vi "View Cooldown Results.vi"(6 "Temperature":dbl, 7 "OSC Configuration":T1(array[cluster]), 9 "Results":dbl[][](array[numeric]), 10 "Lockins":u16[](array[numeric]), 11 "Boolean":bool) -> (3 "Array":cluster{"Y":dbl[], "Y":dbl[]}[][](array[cluster]))   [LabVIEW 2013]
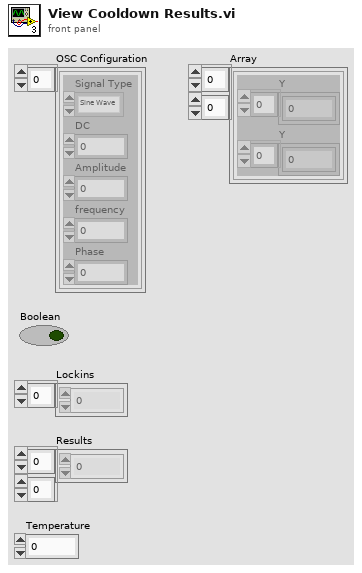
[diagram p1: front panel]
types:
  T1 = cluster{"Signal Type":enum16{"Sine Wave", "Triangle Wave", "Square Wave", "Sawtooth Wave"}, "DC":dbl, "Amplitude":dbl, "frequency":dbl, "Phase":dbl}[]
  T2 = cluster{"Signal Type":enum16{"Sine Wave", "Triangle Wave", "Square Wave", "Sawtooth Wave"}, "DC":dbl, "Amplitude":dbl, "frequency":dbl, "Phase":dbl}
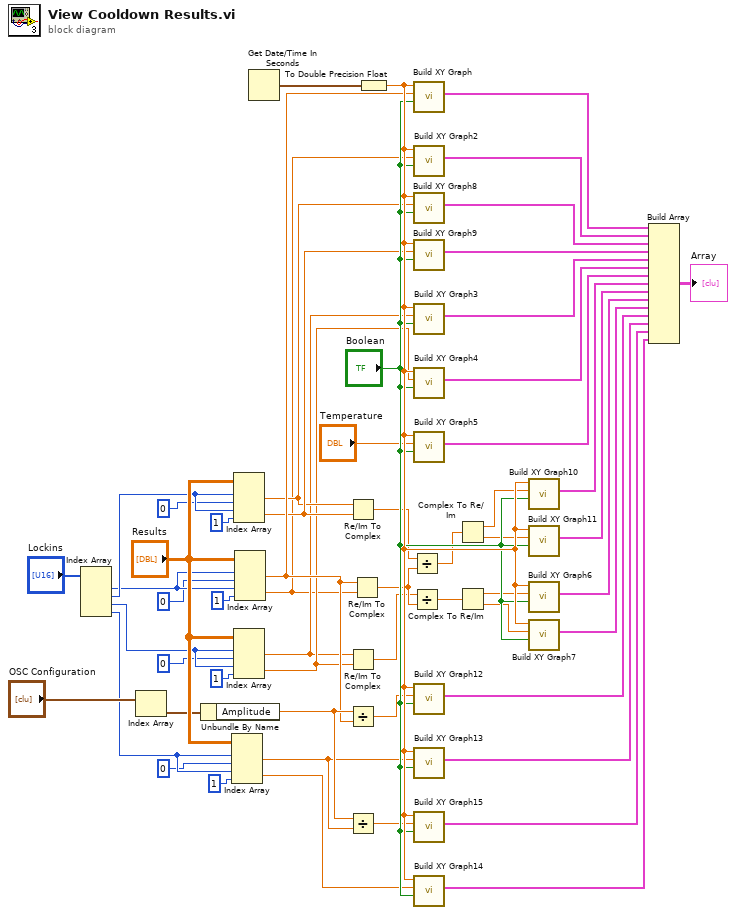
[diagram p0: block diagram]
diagram:
  n1 = Index Array(array="Lockins") -> (element #1=w31:u16, element #2=w32:u16, element #3=w33:u16, element #4=w30:u16)  [unwired: 4 in]
  n2 = Index Array(array="OSC Configuration") -> (element=w37:T2)  [unwired: 1 in]
  n3 = Unbundle By Name(w37) -> ("Amplitude"=w38:dbl)
  n4 = Index Array(array="Results", index (row) #1=w30, index (col) #1=0 ("disabled index (col)"), index (row) #2=w30, index (col) #2=1 ("disabled index (col)")) -> (element #1=w27:dbl, element #2=w26:dbl)
  n5 = Index Array(array="Results", index (row) #1=w32, index (col) #1=0 ("disabled index (col)"), index (row) #2=w32, index (col) #2=1 ("disabled index (col)")) -> (element #1=w15:dbl, element #2=w16:dbl)
  n6 = Index Array(array="Results", index (row) #1=w33, index (col) #1=0 ("disabled index (col)"), index (row) #2=w33, index (col) #2=1 ("disabled index (col)")) -> (element #1=w6:dbl, element #2=w7:dbl)
  n7 = Index Array(array="Results", index (row) #1=w31, index (col) #1=0 ("disabled index (col)"), index (row) #2=w31, index (col) #2=1 ("disabled index (col)")) -> (element #1=w22:dbl, element #2=w5:dbl)
  n8 = Get Date/Time In Seconds() -> (seconds since 1Jan1904=w34:timestamp)
  n9 = Re/Im To Complex(1:w16, 2:w15) -> (0:w17:cdb)
  n10 = Re/Im To Complex(1:w7, 2:w6) -> (0:w8:cdb)
  n11 = Divide(x=w38, y=w22) -> (x/y=w23:dbl)
  n12 = Divide(x=w38, y=w27) -> (x/y=w28:dbl)
  n13 = Re/Im To Complex(1:w5, 2:w22) -> (0:w18:cdb)
  n14 = To Double Precision Float(number=w34) -> (double precision float=w35:dbl)
  n15 = Divide(x=w17, y=w18) -> (x/y=w19:cdb)
  n16 = Divide(x=w8, y=w18) -> (x/y=w9:cdb)
  n17 = call "Build XY Graph"("Reset"="Boolean", "Y Input"=w22, "X Input"=w35) -> ("XY Graph"=w42:cluster{"Y":dbl[], "Y":dbl[]}[])  [unwired: 2 in, 6 out]
  n18 = call "Build XY Graph2"("Reset"="Boolean", "Y Input"=w5, "X Input"=w35) -> ("XY Graph"=w43:cluster{"Y":dbl[], "Y":dbl[]}[])  [unwired: 2 in, 6 out]
  n19 = call "Build XY Graph8"("Reset"="Boolean", "Y Input"=w15, "X Input"=w35) -> ("XY Graph"=w44:cluster{"Y":dbl[], "Y":dbl[]}[])  [unwired: 2 in, 6 out]
  n20 = call "Build XY Graph9"("Reset"="Boolean", "Y Input"=w16, "X Input"=w35) -> ("XY Graph"=w45:cluster{"Y":dbl[], "Y":dbl[]}[])  [unwired: 2 in, 6 out]
  n21 = call "Build XY Graph3"("Reset"="Boolean", "Y Input"=w6, "X Input"=w35) -> ("XY Graph"=w46:cluster{"Y":dbl[], "Y":dbl[]}[])  [unwired: 2 in, 6 out]
  n22 = call "Build XY Graph4"("Reset"="Boolean", "Y Input"=w7, "X Input"=w35) -> ("XY Graph"=w47:cluster{"Y":dbl[], "Y":dbl[]}[])  [unwired: 2 in, 6 out]
  n23 = call "Build XY Graph5"("Reset"="Boolean", "Y Input"="Temperature", "X Input"=w35) -> ("XY Graph"=w48:cluster{"Y":dbl[], "Y":dbl[]}[])  [unwired: 2 in, 6 out]
  n24 = call "Build XY Graph12"("Reset"="Boolean", "Y Input"=w23, "X Input"=w35) -> ("XY Graph"=w51:cluster{"Y":dbl[], "Y":dbl[]}[])  [unwired: 2 in, 6 out]
  n25 = call "Build XY Graph13"("Reset"="Boolean", "Y Input"=w27, "X Input"=w35) -> ("XY Graph"=w54:cluster{"Y":dbl[], "Y":dbl[]}[])  [unwired: 2 in, 6 out]
  n26 = call "Build XY Graph15"("Reset"="Boolean", "Y Input"=w28, "X Input"=w35) -> ("XY Graph"=w55:cluster{"Y":dbl[], "Y":dbl[]}[])  [unwired: 2 in, 6 out]
  n27 = call "Build XY Graph14"("Reset"="Boolean", "Y Input"=w26, "X Input"=w35) -> ("XY Graph"=w56:cluster{"Y":dbl[], "Y":dbl[]}[])  [unwired: 2 in, 6 out]
  n28 = Complex To Re/Im(x + iy=w19) -> (x=w20:dbl, y=w21:dbl)
  n29 = Complex To Re/Im(x + iy=w9) -> (x=w11:dbl, y=w10:dbl)
  n30 = call "Build XY Graph10"("Reset"="Boolean", "Y Input"=w20, "X Input"=w35) -> ("XY Graph"=w49:cluster{"Y":dbl[], "Y":dbl[]}[])  [unwired: 2 in, 6 out]
  n31 = call "Build XY Graph11"("Reset"="Boolean", "Y Input"=w21, "X Input"=w35) -> ("XY Graph"=w50:cluster{"Y":dbl[], "Y":dbl[]}[])  [unwired: 2 in, 6 out]
  n32 = call "Build XY Graph6"("Reset"="Boolean", "Y Input"=w11, "X Input"=w35) -> ("XY Graph"=w52:cluster{"Y":dbl[], "Y":dbl[]}[])  [unwired: 2 in, 6 out]
  n33 = call "Build XY Graph7"("Reset"="Boolean", "Y Input"=w10, "X Input"=w35) -> ("XY Graph"=w53:cluster{"Y":dbl[], "Y":dbl[]}[])  [unwired: 2 in, 6 out]
  n34 = Build Array(w42, w43, w44, w45, w46, w47, w48, w49, w50, w52, w53, w51, w54, w55, w56) -> (→"Array":cluster{"Y":dbl[], "Y":dbl[]}[][])
